vi "Mcp2210 Get Library Version.vi"(8 "error in (no error)":errorcluster) -> (0 "error out":errorcluster, 3 "version":string)   [LabVIEW 2015, in "mcp2210.lvlib"]
doc: "Provides the library version as NULL terminated UNICODE string.\nParameters:\nInputs:\n- none\nOutputs:\n- wchar_t *version - Pointer to buffer string of 64 bytes (MPC2210_LIBRARY_VERSION_SIZE) in size\n(So it can accommodate max 30 wide characters.)\nThe version string, including the NULL terminator is copied in this buffer.\nCannot be NULL.\nReturns:\n- positive value: version string size (bytes) including the null character\n- negative value: E_ERR_NULL (-10) if *version is NULL\n\nMCP2210_DLL_UM_API int __stdcall Mcp2210_GetLibraryVersion(unsigned short *version);"
uses:
  <userlib>/mcp2210/mcp2210.lvlib
  <userlib>/mcp2210/mcp2210_dll_um_x86.dll
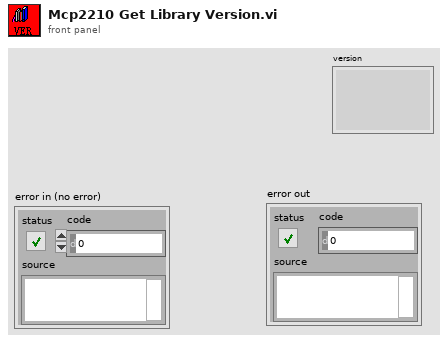
[diagram p1: front panel]
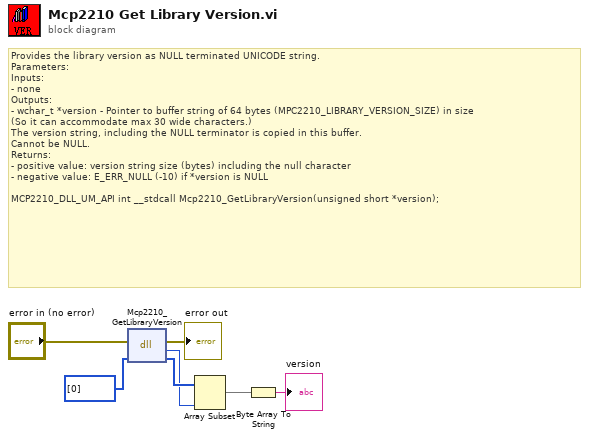
[diagram p0: block diagram]
diagram:
  # "Provides the library version as NULL terminated UNICODE string.\nParameters:\nInputs:\n- none\nOutputs:\n- wchar_t *version - Pointer to buffer string of 64 bytes (MPC2210_LIBRARY_VERSION_SIZE) in size\n(So it can accommodate max 30 wide characters.)\nThe version string, including the NULL terminator is copied in this buffer.\nCannot be NULL.\nReturns:\n- positive value: version string size (bytes) including the null character\n- negative value: E_ERR_NULL (-10) if *version is NULL\n\nMCP2210_DLL_UM_API int __stdcall Mcp2210_GetLibraryVersion(unsigned short *version);"
  n1 = dll-call lib="D:/LabVIEW 2015/user.lib/mcp2210/mcp2210_dll_um_x86.*" fn="Mcp2210_GetLibraryVersion"(error in="error in (no error)", "version"=u16[] [0]) -> (error out=→"error out":errorcluster, "return type"=w5:i32, "version"=w6:u16[])  [unwired: 2 in, 1 out]
  n2 = Array Subset(array=w6, length=w5) -> (w4:u16[])  [unwired: 1 in]
  n3 = Byte Array To String(unsigned byte array=w4) -> (string=→"version":string)
